vi "ATF-Pump-RPM_Module_A.vi"(7 "Data FIFO Ref":T1, 8 "error in (no error)":errorcluster, 11 "TCP Network Connection in":refnum<k5>) -> (0 "error out":errorcluster, 3 "TCP Network Connection out":refnum<k5>)   [LabVIEW 2022 SP3]
uses:
  RT Controls/ATF-Pump-Data FIFO.ctl
  RT Controls/ATF-Pump-FGV Read write.ctl
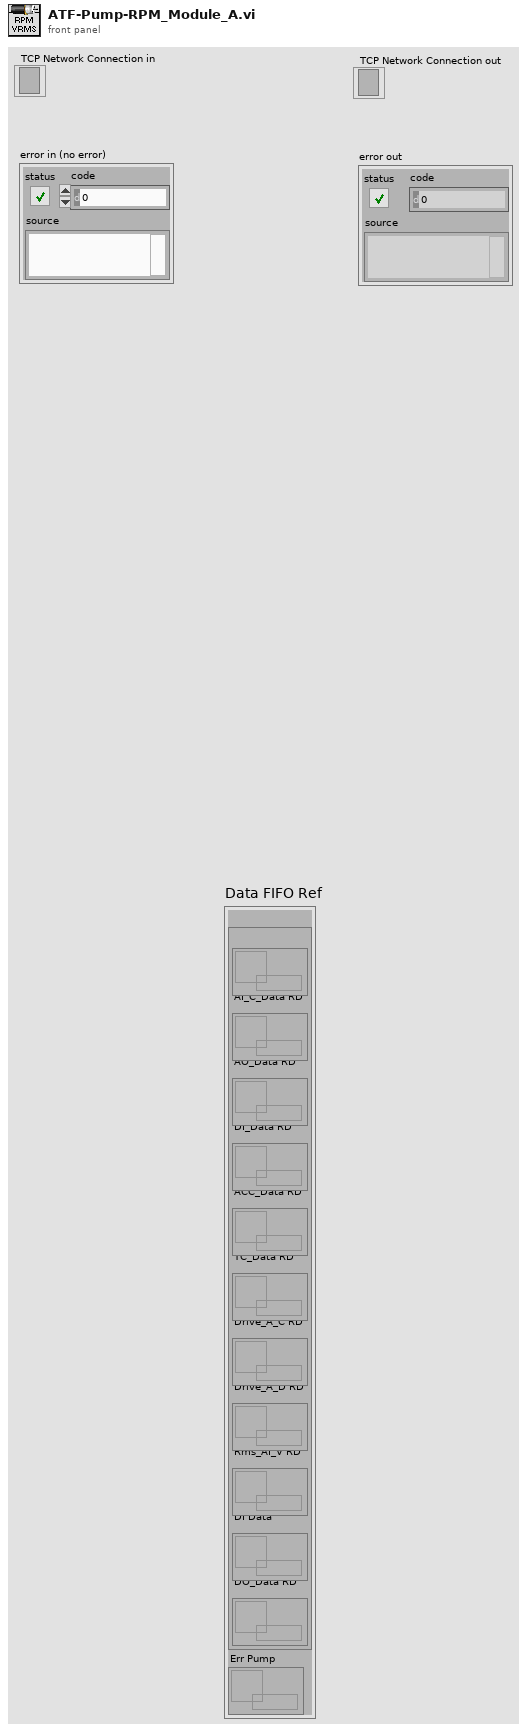
[diagram p1: front panel]
types:
  T1 = typedef "ATF-Pump-Data FIFO.ctl" = cluster{"RD":cluster{"AI_V_Data RD":refnum<queue>, "AI_C_Data RD":refnum<queue>, "AO_Data RD":refnum<queue>, "DI_Data RD":refnum<queue>, "ACC_Data RD":refnum<queue>, "TC_Data RD":refnum<queue>, "Drive_A_C RD":refnum<queue>, "Drive_A_D RD":refnum<queue>, "Rms_AI_V RD":refnum<queue>, "DI Data":refnum<queue>, "DO_Data RD":refnum<queue>}, "Err Pump":refnum<queue>}
  T2 = typedef "ATF-Pump-FGV Read write.ctl" = enum16{"Write", "Read"}
  T3 = cluster{"En_Drive_A":bool, "En_Drive_L":bool, "Exit_Drive_A":bool, "Exit_Drive_L":bool}
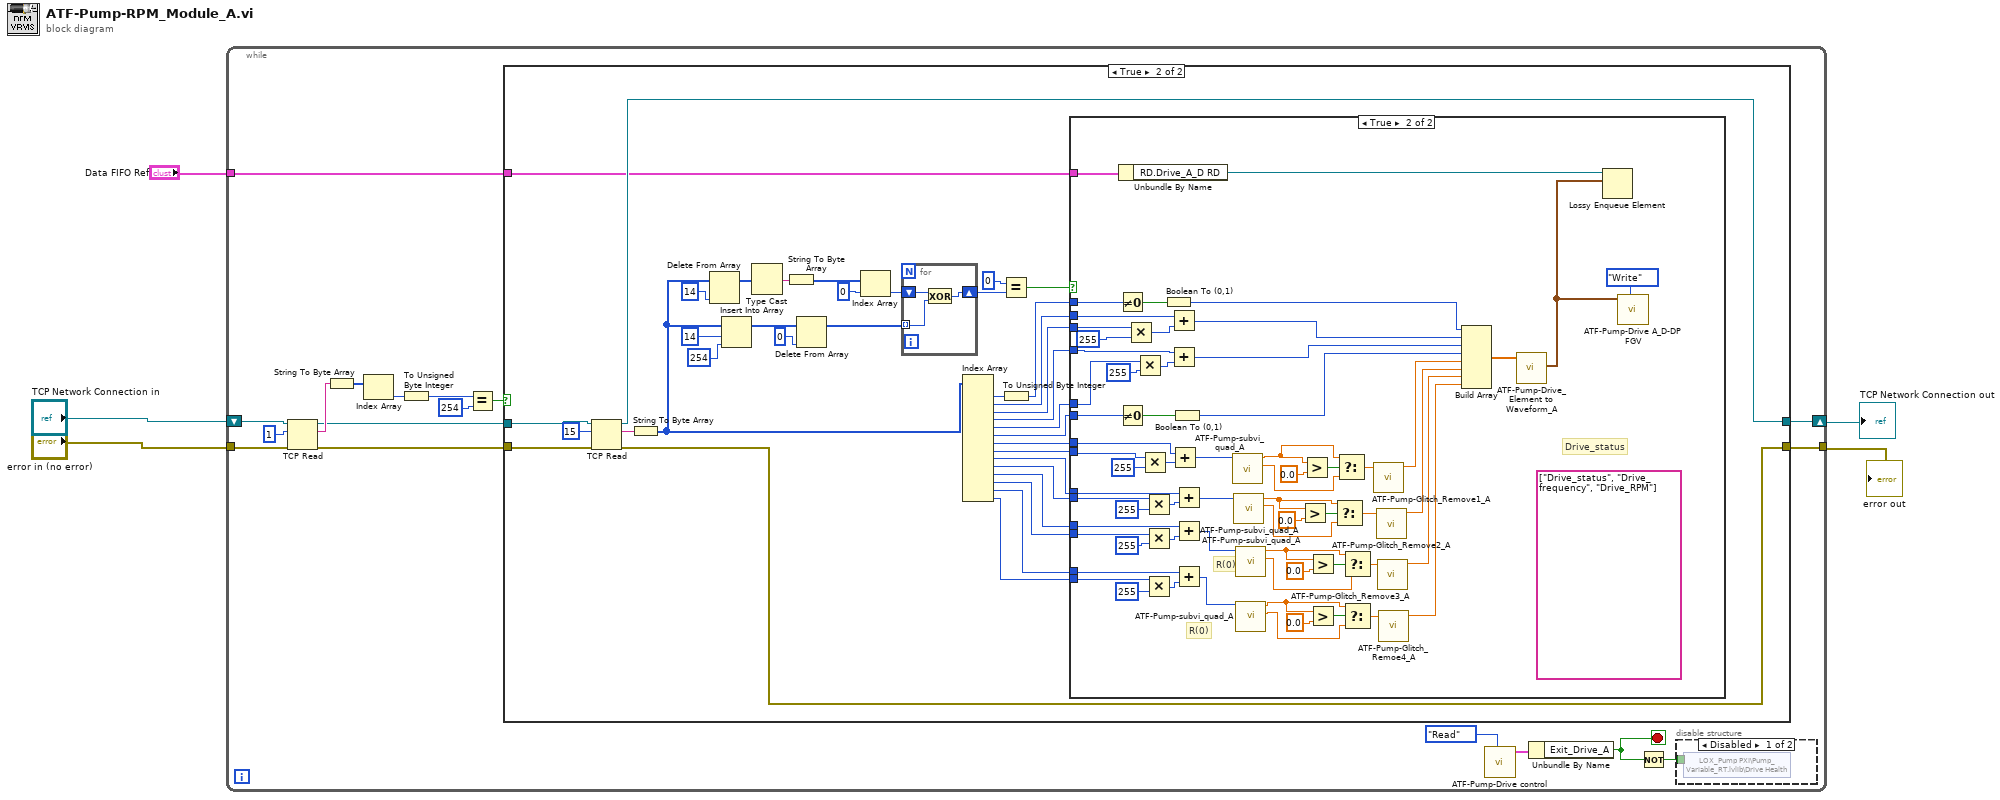
[diagram p0: block diagram]
diagram:
  n1 = while {
    tunnel: "error in (no error)" -> [w22]
    shift-right: [w11] -> w5
    shift-left: "TCP Network Connection in" -> [w23]
    tunnel: [w12] -> w4
    tunnel: "Data FIFO Ref" -> [w6]
    stop <- w7 stop-if-true
    n2 = TCP Read(connection ID=w23, bytes to read=1, error in (no error)=w22) -> (connection ID out=w15:refnum<k5>, data out=w21:string, error out=w14:errorcluster)  [unwired: 2 in]
    n3 = String To Byte Array(string=w21) -> (unsigned byte array=w20:u8[])
    n4 = Index Array(array=w20) -> (element=w19:u8)  [unwired: 1 in]
    n5 = To Unsigned Byte Integer(number=w19) -> (unsigned 8bit integer=w18:u8)
    n6 = Equal?(x=w18, y=u8 254) -> (x = y?=w16:bool)
    n7 = case shown="True" w16 {
      tunnel: w15 -> [w26 w63]
      tunnel: w14 -> [w25 w62]
      tunnel: [w26 w52] -> w11
      tunnel: [w25 w37] -> w12
      tunnel: w6 -> [_ w27]
      frame False {
      }
      frame True {
        n8 = TCP Read(connection ID=w63, bytes to read=15, error in (no error)=w62) -> (connection ID out=w52:refnum<k5>, data out=w60:string, error out=w37:errorcluster)  [unwired: 2 in]
        n9 = String To Byte Array(string=w60) -> (unsigned byte array=w45:u8[])
        n10 = Delete From Array(array=w45, index=14) -> (array with subset deleted=w58:u8[])  [unwired: 1 in, 1 out]
        n11 = Insert Into Array(array=w45, index=14, new element=u8 254 ("new element/subarray")) -> (w51:u8[])
        n12 = Type Cast(x=w58) -> (*(type *) &x=w57:string)  [unwired: 1 in]
        n13 = String To Byte Array(string=w57) -> (unsigned byte array=w56:u8[])
        n14 = Delete From Array(array=w51, index=0) -> (array with subset deleted=w48:u8[])  [unwired: 1 in, 1 out]
        n15 = Index Array(array=w56, index=0) -> (element=w49:u8)
        n16 = for {
          shift-right: [w130] -> w47
          shift-left: w49 -> [w131]
          tunnel: w48 -> [w129] mode=indexing
          n17 = Exclusive Or(1:w129, 2:w131) -> (0:w130:u8)
        }
        n18 = Index Array(array=w45) -> (element #1=w44:u8, element #2=w42:u8, element #3=w41:u8, element #4=w40:u8, element #5=w39:u8, element #6=w38:u8, element #7=w35:u8, element #8=w34:u8, element #9=w33:u8, element #10=w32:u8, element #11=w31:u8, element #12=w30:u8, element #13=w29:u8, element #14=w28:u8)  [unwired: 14 in]
        n19 = Equal?(x=u8 0, y=w47) -> (x = y?=w46:bool)
        n20 = To Unsigned Byte Integer(number=w44) -> (unsigned 8bit integer=w43:u8)
        n21 = case shown="True" w46 {
          tunnel: w43 -> [_ w128]
          tunnel: w42 -> [_ w96]
          tunnel: w41 -> [_ w95]
          tunnel: w40 -> [_ w94]
          tunnel: w39 -> [_ w93]
          tunnel: w38 -> [_ w124]
          tunnel: w35 -> [_ w115]
          tunnel: w34 -> [_ w114]
          tunnel: w33 -> [_ w113]
          tunnel: w32 -> [_ w112]
          tunnel: w31 -> [_ w111]
          tunnel: w30 -> [_ w110]
          tunnel: w29 -> [_ w109]
          tunnel: w28 -> [_ w108]
          tunnel: w27 -> [_ w67]
          frame False {
          }
          frame True {
            (unwired) string[] ["Drive_status", "Drive_frequency", "Drive_RPM"]
            # "Drive_status"
            # "R(0)"
            # "R(0)"
            n22 = Not Equal To 0?(x=w128) -> (x != 0?=w99:bool)
            n23 = Not Equal To 0?(x=w124) -> (x != 0?=w98:bool)
            n24 = Unbundle By Name(w67) -> ("RD.Drive_A_D RD"=w66:refnum<queue>)
            n25 = Multiply(x=w95, y=u32 255) -> (x*y=w97:u32)
            n26 = Multiply(x=w93, y=u32 255) -> (x*y=w125:u32)
            n27 = Multiply(x=w114, y=u32 255) -> (x*y=w116:u32)
            n28 = Multiply(x=w112, y=u32 255) -> (x*y=w119:u32)
            n29 = Multiply(x=w110, y=u32 255) -> (x*y=w120:u32)
            n30 = Multiply(x=w108, y=u32 255) -> (x*y=w123:u32)
            n31 = Boolean To (0,1)(Boolean=w99) -> (0, 1=w92:i16)
            n32 = Add(x=w96, y=w97) -> (x+y=w91:u32)
            n33 = Add(x=w94, y=w125) -> (x+y=w90:u32)
            n34 = Add(x=w115, y=w116) -> (x+y=w88:u32)
            n35 = Boolean To (0,1)(Boolean=w98) -> (0, 1=w89:i16)
            n36 = Add(x=w113, y=w119) -> (x+y=w85:u32)
            n37 = Add(x=w111, y=w120) -> (x+y=w82:u32)
            n38 = Add(x=w109, y=w123) -> (x+y=w79:u32)
            n39 = call "ATF-Pump-subvi_quad_A.vi"("input variable"=w88) -> ("output variable 2"=w86:dbl, "output variable"=w87:dbl)  [unwired: 8 in]
            n40 = call "ATF-Pump-subvi_quad_A.vi"("input variable"=w85) -> ("output variable 2"=w83:dbl, "output variable"=w84:dbl)  [unwired: 8 in]
            n41 = call "ATF-Pump-subvi_quad_A.vi"("input variable"=w82) -> ("output variable 2"=w80:dbl, "output variable"=w81:dbl)  [unwired: 8 in]
            n42 = call "ATF-Pump-subvi_quad_A.vi"("input variable"=w79) -> ("output variable 2"=w77:dbl, "output variable"=w78:dbl)  [unwired: 8 in]
            n43 = Greater?(x=w84, y=0.0) -> (0:w102:bool)
            n44 = Greater?(x=w87, y=0.0) -> (0:w100:bool)
            n45 = Greater?(x=w81, y=0.0) -> (0:w104:bool)
            n46 = Greater?(x=w78, y=0.0) -> (0:w106:bool)
            n47 = Select(t=w84, s=w102, f=w83) -> (s? t:f=w70:dbl)
            n48 = Select(t=w87, s=w100, f=w86) -> (s? t:f=w76:dbl)
            n49 = Select(t=w81, s=w104, f=w80) -> (s? t:f=w72:dbl)
            n50 = Select(t=w78, s=w106, f=w77) -> (s? t:f=w74:dbl)
            n51 = call "ATF-Pump-Glitch_Remove1_A.vi"("Input"=w76) -> ("Output"=w75:dbl)  [unwired: 10 in]
            n52 = call "ATF-Pump-Glitch_Remove2_A.vi"("Input"=w70) -> ("Output"=w69:dbl)  [unwired: 10 in]
            n53 = call "ATF-Pump-Glitch_Remove3_A.vi"("Input"=w72) -> ("Output"=w71:dbl)  [unwired: 10 in]
            n54 = call "ATF-Pump-Glitch_Remoe4_A.vi"("Input"=w74) -> ("Output"=w73:dbl)  [unwired: 10 in]
            n55 = Build Array(w92, w91, w90, w89, w75, w69, w71, w73) -> (w68:dbl[])
            n56 = call "ATF-Pump-Drive_Element to Waveform_A.vi"("Array input"=w68) -> ("RPM out"=w65:waveform(dbl)[])  [unwired: 10 in]
            n57 = Lossy Enqueue Element(queue=w66, element=w65) -> ()  [unwired: 1 in, 4 out]
            n58 = call "ATF-Pump-Drive A_D-DP FGV.vi"("Write/Read"=ATF-Pump-FGV_Read_write."Write", "Drive A_D"=w65) -> ()  [unwired: 8 in, 2 out]
          }
        }
      }
    }
    n59 = call "ATF-Pump-Drive control.vi"("Action"=enum16{"Init", "Write", "Read"}."Read") -> ("Loop Control Out"=w8:T3)  [unwired: 9 in, 1 out]
    n60 = Unbundle By Name(w8) -> ("Exit_Drive_A"=w7:bool)
    n61 = Not(x=w7) -> (.not. x?=w10:bool)
    n62 = disable-structure shown="Disabled" {
      disable-tunnel: w10 -> [w24 _]
      frame Disabled {
        n63 = shared-variable "LOX_Pump PXI\\Pump_Variable_RT.lvlib\\Drive Health"(w24) -> ()  [unwired: 1 in, 1 out]
      }
      frame Enabled {
      }
    }
  }
  "TCP Network Connection out" <- w5
  "error out" <- w4
